vi "Read Decimal Places.vi"(7 "Unit ID (A)":string="A", 8 "error in":errorcluster, 10 "Software Version":u8, 11 "VISA Session In":refnum<visa-resource-name>="Alicat") -> (0 "error out":errorcluster, 2 "Decimal places":T1, 3 "VISA Session Out":refnum<visa-resource-name>)   [LabVIEW 2015]
doc: "Reads the decimal places of the pressure and flow rate variables."
uses:
  <vilib>/Instr/_visa.llb/VISA Flush IO Buffer Mask.ctl
panel:
  # "SW Version defaults to 0. \nIf un-wired, it will call a \nsub-VI to check."
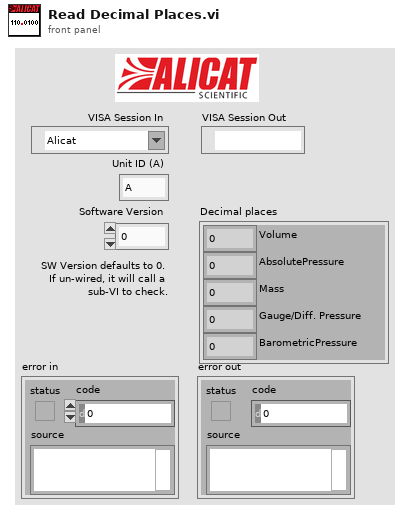
[diagram p1: front panel]
types:
  T1 = cluster{"Volume":i32, "AbsolutePressure":i32, "Mass":i32, "Gauge/Diff. Pressure":i32, "BarometricPressure":i32}
  T2 = typedef "VISA Flush IO Buffer Mask.ctl" = u16
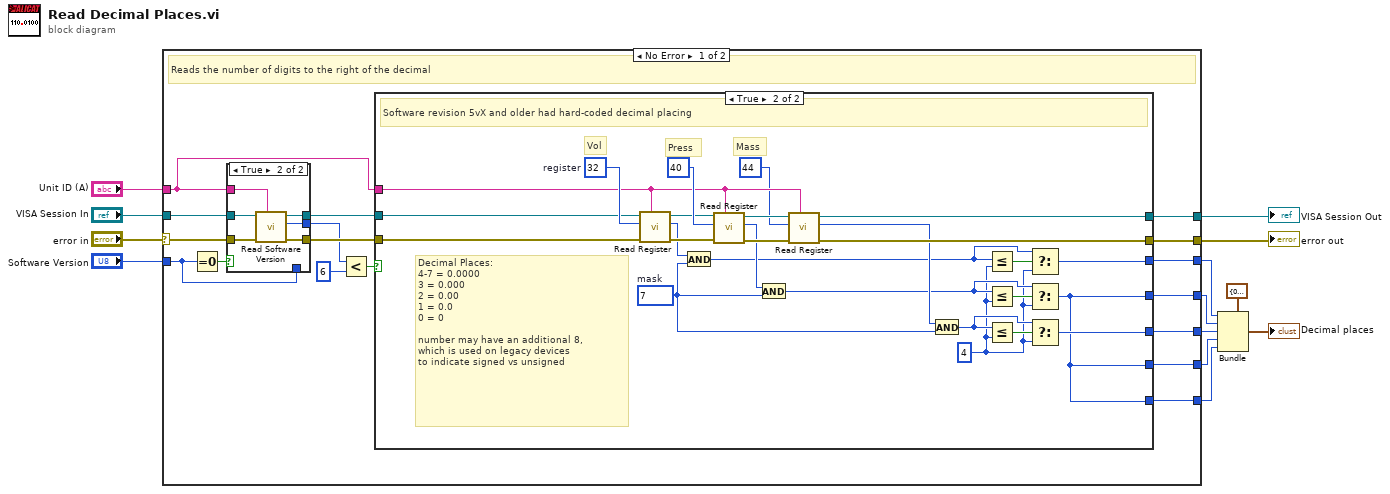
[diagram p0: block diagram]
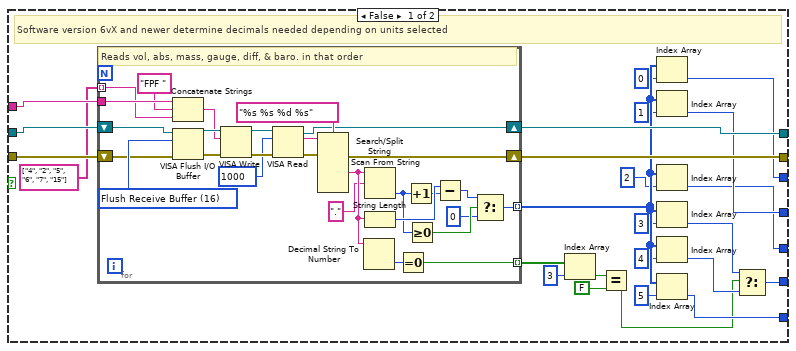
[diagram p3: hidden frame]
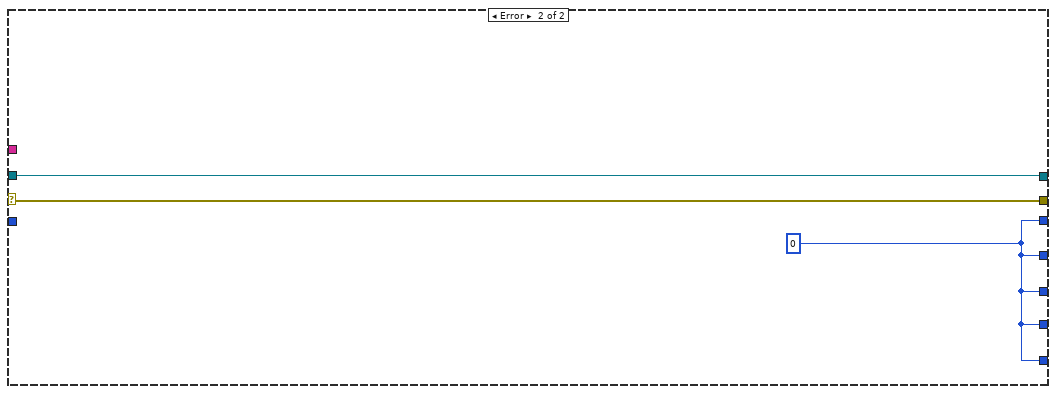
[diagram p4: hidden frame]
diagram:
  n1 = case shown="No Error" "error in" {
    selector: "error in" -> [w25 w120]
    tunnel: "VISA Session In" -> [w24 w121]
    tunnel: "Unit ID (A)" -> [w23 _]
    tunnel: [w30 w121] -> w11
    tunnel: [w29 w120] -> w10
    tunnel: [w28 w119] -> w5
    tunnel: [w27 w119] -> w4
    tunnel: [w26 w119] -> w3
    tunnel: [w17 w119] -> w2
    tunnel: [w16 w119] -> w1
    tunnel: "Software Version" -> [w14 _]
    frame No Error {
      # "Reads the number of digits to the right of the decimal"
      n2 = Equal To 0?(x=w14) -> (x = 0?=w15:bool)
      n3 = case shown="True" w15 {
        tunnel: w25 -> [w32 w39]
        tunnel: w24 -> [w31 w38]
        tunnel: w23 -> [_ w37]
        tunnel: [w32 w36] -> w22
        tunnel: [w31 w35] -> w21
        tunnel: [w33 w34] -> w20
        tunnel: w14 -> [w33 _]
        frame False {
        }
        frame True {
          n4 = call "Read Software Version.vi"("Unit ID (A)"=w37, "error in"=w39, "VISA Session In"=w38) -> ("error out"=w36:errorcluster, "Software Version"=w34:u8, "VISA Session Out"=w35:refnum<visa-resource-name>)  [unwired: 6 in]
        }
      }
      n5 = Less?(x=w20, y=u8 6) -> (x < y?=w19:bool)
      n6 = case shown="True" w19 {
        tunnel: w21 -> [w63 w117]
        tunnel: w23 -> [w62 w114]
        tunnel: [w60 w110] -> w30
        tunnel: [w61 w109] -> w29
        tunnel: w22 -> [w64 w103]
        tunnel: [w50 w102] -> w28
        tunnel: [w49 w93] -> w27
        tunnel: [w48 w98] -> w26
        tunnel: [w54 w93] -> w17
        tunnel: [w51 w93] -> w16
        frame False {
          # "Software version 6vX and newer determine decimals needed depending on units selected"
          n7 = for {
            tunnel: w62 -> [w82]
            shift-right: [w79] -> w61
            shift-left: w64 -> [w88]
            shift-right: [w78] -> w60
            shift-left: w63 -> [w87]
            tunnel: string[] ["4", "2", "5", "6", "7", "15"] ("appended array") -> [w76] mode=indexing
            tunnel: [w68] -> w47 mode=indexing
            tunnel: [w73] -> w58 mode=indexing
            w91 = T2 16 items=["Flush Receive Buffer"=16, "Write Transmit Buffer to Device"=32, "Flush Receive Buffer (No I/O)"=64, "Flush Transmit Buffer"=128] ("Mask")
            # "Reads vol, abs, mass, gauge, diff, & baro. in that order"
            n8 = Concatenate Strings(w82, "FPF " ("format string (polled)"), w76) -> (w77:string)
            n9 = VISA Flush I/O Buffer(VISA resource name=w87, mask (16)=w91, error in (no error)=w88) -> (VISA resource name out=w84:refnum<visa-resource-name>, error out=w83:errorcluster)
            n10 = VISA Write(VISA resource name=w84, write buffer=w77, error in (no error)=w83) -> (VISA resource name out=w90:refnum<visa-resource-name>, error out=w92:errorcluster)  [unwired: 1 out]
            n11 = VISA Read(VISA resource name=w90, byte count=u32 1000, error in (no error)=w92) -> (VISA resource name out=w78:refnum<visa-resource-name>, read buffer=w85:string, error out=w80:errorcluster)  [unwired: 1 out]
            n12 = Scan From String(format string="%s %s %d %s", input string=w85, error in=w80) -> (error out=w79:errorcluster, output 2=w72:string)  [unwired: 8 in, 2 out]
            n13 = Decimal String To Number(string=w72) -> (number=w74:i32)  [unwired: 2 in, 1 out]
            n14 = Search/Split String(string=w72, search string/char (-)="." ("regular expression")) -> (offset of match=w69:i32)  [unwired: 1 in, 2 out]
            n15 = String Length(string=w72) -> (length=w75:i32)
            n16 = Equal To 0?(x=w74) -> (x = 0?=w73:bool)
            n17 = Increment(x=w69) -> (x+1=w70:i32)
            n18 = Greater Or Equal To 0?(x=w69) -> (x >= 0?=w66:bool)
            n19 = Subtract(x=w75, y=w70) -> (x-y=w67:i32)
            n20 = Select(t=w67, s=w66, f=0) -> (s? t:f=w68:i32)
          }
          n21 = Index Array(array=w58, index=3) -> (element=w56:bool)
          n22 = Equal?(x=w56, y=FALSE) -> (x = y?=w40:bool)
          n23 = Index Array(array=w47, index=0) -> (element=w50:i32)
          n24 = Index Array(array=w47, index=1) -> (element=w49:i32)
          n25 = Index Array(array=w47, index=2) -> (element=w48:i32)
          n26 = Index Array(array=w47, index=3) -> (element=w53:i32)
          n27 = Index Array(array=w47, index=4) -> (element=w52:i32)
          n28 = Index Array(array=w47, index=5) -> (element=w51:i32)
          n29 = Select(t=w53, s=w40, f=w52) -> (s? t:f=w54:i32)
        }
        frame True {
          w94 = 4 ("y")
          w104 = 7  # mask
          w118 = u16 32  # register
          # "Decimal Places:\n4-7 = 0.0000\n3 = 0.000\n2 = 0.00\n1 = 0.0\n0 = 0\n\nnumber may have an additional 8,\nwhich is used on legacy devices \nto indicate signed vs unsigned"
          # "Mass"
          # "Press"
          # "Vol"
          # "Software revision 5vX and older had hard-coded decimal placing"
          n30 = call "Read Register.vi"("Unit ID (A)"=w114, "error in"=w103, "Register address"=w118, "VISA Session In"=w117) -> ("error out"=w113:errorcluster, "Register Value (I32)"=w107:i32, "VISA Session Out"=w115:refnum<visa-resource-name>)  [unwired: 5 in]
          n31 = And(x=w107, y=w104) -> (x .and. y?=w95:i32)
          n32 = call "Read Register.vi"("Unit ID (A)"=w114, "error in"=w113, "Register address"=u16 40, "VISA Session In"=w115) -> ("error out"=w112:errorcluster, "Register Value (I32)"=w105:i32, "VISA Session Out"=w111:refnum<visa-resource-name>)  [unwired: 5 in]
          n33 = And(x=w105, y=w104) -> (x .and. y?=w96:i32)
          n34 = call "Read Register.vi"("Unit ID (A)"=w114, "error in"=w112, "Register address"=u16 44, "VISA Session In"=w111) -> ("error out"=w109:errorcluster, "Register Value (I32)"=w106:i32, "VISA Session Out"=w110:refnum<visa-resource-name>)  [unwired: 5 in]
          n35 = And(x=w106, y=w104) -> (x .and. y?=w97:i32)
          n36 = Less Or Equal?(x=w95, y=w94) -> (x <= y?=w101:bool)
          n37 = Less Or Equal?(x=w96, y=w94) -> (x <= y?=w100:bool)
          n38 = Less Or Equal?(x=w97, y=w94) -> (x <= y?=w99:bool)
          n39 = Select(t=w95, s=w101, f=w94) -> (s? t:f=w102:i32)
          n40 = Select(t=w96, s=w100, f=w94) -> (s? t:f=w93:i32)
          n41 = Select(t=w97, s=w99, f=w94) -> (s? t:f=w98:i32)
        }
      }
    }
    frame Error {
      w119 = 0
    }
  }
  "error out" <- w10
  "VISA Session Out" <- w11
  n42 = Bundle(cluster=T1 {"Volume"=0, "AbsolutePressure"=0, "Mass"=0, "Gauge/Diff. Pressure"=0, "BarometricPressure"=0} ("output cluster"), "Volume"=w5, "AbsolutePressure"=w4, "Mass"=w3, "Gauge/Diff. Pressure"=w2, "BarometricPressure"=w1) -> (→"Decimal places":T1)
